vi "quit.vi"(8 "error in (no error)":errorcluster, 11 "canon_m3 in":refnum<class "protocol_canonM3.lvclass">) -> (0 "error out":errorcluster, 3 "canon_m3 out":refnum<class "protocol_canonM3.lvclass">)   [LabVIEW 2015, in "protocol_canonM3.lvclass"]
uses:
  protocol_canonM3.lvclass
  protocol_canonM3.lvclass/protocol_canonM3.ctl
  protocol_Generic/Protocol_Generic.lvclass
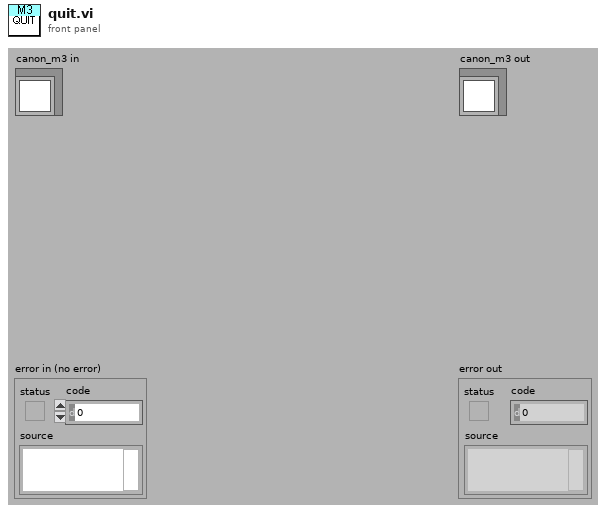
[diagram p1: front panel]
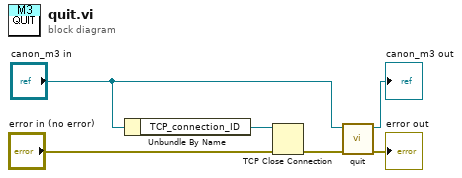
[diagram p0: block diagram]
diagram:
  n1 = Unbundle By Name("canon_m3 in") -> ("TCP_connection_ID"=w1:refnum<k5>)
  n2 = TCP Close Connection(connection ID=w1, error in (no error)="error in (no error)") -> (error out=w3:errorcluster)  [unwired: 1 in, 1 out]
  n3 = call-parent "quit.vi"("error in (no error)"=w3, "Protocol_Generic in"="canon_m3 in") -> ("error out"=→"error out":errorcluster, "Protocol_Generic out"=→"canon_m3 out":refnum<class "protocol_canonM3.lvclass">)  [unwired: 8 in]
